vi "Init AP Sx Object.vi"(6 "otpOffset":i32, 7 "otpCurrent":i32, 8 "error in (no error)":errorcluster caption="错误输入（无错误）", 9 "outCurrent":i32, 10 "asicType":i32, 11 "asicHandle":i32) -> (0 "error out":errorcluster caption="错误输出", 3 "function return":i32)   [LabVIEW 2020]
doc: "extern int __stdcall InitAPSxObject (int asicHandle, IN int asicType, IN int outCurrent, IN int otpCurrent, IN int otpOffset);"
uses:
  APSx.dll/APSx.dll
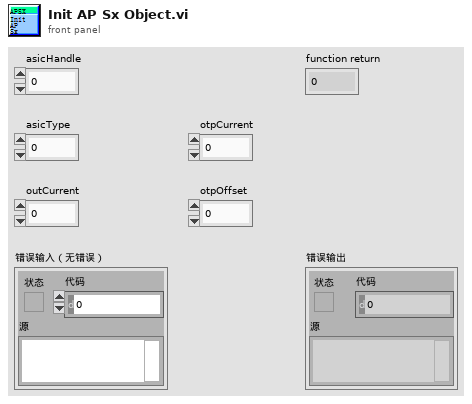
[diagram p1: front panel]
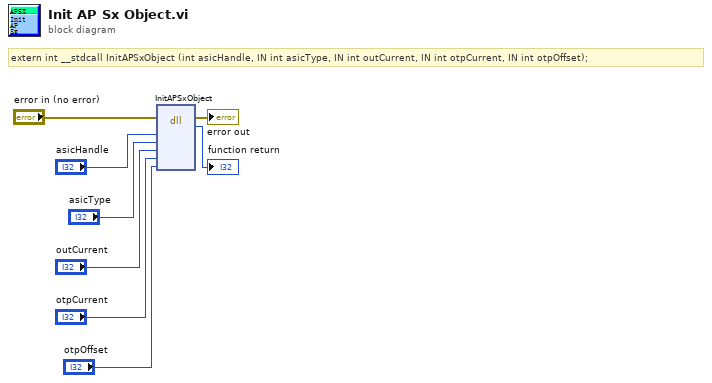
[diagram p0: block diagram]
diagram:
  # "extern int __stdcall InitAPSxObject (int asicHandle, IN int asicType, IN int outCurrent, IN int otpCurrent, IN int otpOffset);"
  n1 = dll-call lib="PTH2iabs CUsersFengDesktop传感器对中台传感器对中台labviewSourcesAPSx.dllAPSx.dll" fn="InitAPSxObject"(error in="error in (no error)", "asicHandle"="asicHandle", "asicType"="asicType", "outCurrent"="outCurrent", "otpCurrent"="otpCurrent", "otpOffset"="otpOffset") -> (error out=→"error out":errorcluster, "返回类型"=→"function return":i32)  [unwired: 7 in, 1 out]
